vi "Triggering.vi"(11 "Test Case In":refnum<class "Test.Camera.lvclass">) -> (0 "error out":errorcluster, 3 "Test Case Out":refnum<class "Test.Camera.lvclass">)   [LabVIEW 2020, in "Test.Camera.lvclass"]
uses:
  Test.Camera.lvclass
  C:/Program Files (x86)/National Instruments/LabVIEW 2020/vi.lib/Astemes/LUnit/Test Case.lvclass
  g_industrial_cam/Camera/Camera.lvclass/Camera.ctl
  <vilib>/Astemes/LUnit/Test Case.lvclass/Test Case.ctl
  g_industrial_cam/Buffer/Buffer.lvclass/Buffer.ctl
  c3e2611f-c54f-4219-a549-b8da21c7f085.vi
  48e9c757-fedc-43ef-b150-82f816eea71f.vi
  6c7b76fd-512f-40e9-9fec-d585849d84ab.vi
  g_industrial_cam/Camera/GetSetTrigger.vi
  <vilib>/Astemes/LUnit/Append Pass Result.vi
  <vilib>/Astemes/LUnit/Append Fail Result.vi
  Get Alternative List Value.vi/1a5b698b-b1e6-4ec2-a46b-3d59f4d11909.vi
  <vilib>/Astemes/LUnit/Describe Comparison.vi
  48e9c757-fedc-43ef-b150-82f816eea71f.vi/9c5d11cd-9439-4240-a1ee-d9baace9c924.vi
  g_industrial_cam/Buffer/Access Handle.vi
  <vilib>/Astemes/LUnit/Run In UI.vi
  <vilib>/Utility/error.llb/Clear Errors.vi
  g_industrial_cam/Camera/Check Not Disconnected.vi
  <vilib>/Utility/error.llb/Error Cluster From Error Code.vi
  <vilib>/Astemes/LUnit/Describe Variant.vi
  g_industrial_cam/Camera/Destroy Stream Events.vi
  g_industrial_cam/Camera/Check Stream OK.vi
  <vilib>/Comparison/Equal/Equal Functor/Equal Functor.lvclass
  g_industrial_cam/Buffer/Buffer.lvclass
  Test.Camera.lvclass/Test.Camera.ctl
  <vilib>/Astemes/LUnit/Test Case.lvclass
  g_industrial_cam/Camera/Camera.lvclass
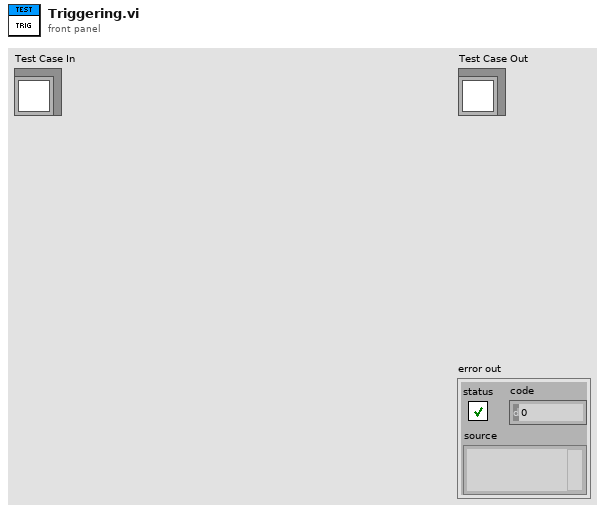
[diagram p1: front panel]
types:
  T1 = enum16{"Get Values", "Configure Trigger", "Software Trigger"}
  T2 = enum16{"Get Values", "Configure Trigger", "Software Trigger"}[]
  T3 = cluster{"Trigger Source":string, "Supported":bool, "Available Triggers":string[], "Available Trigger Sources":string[]}
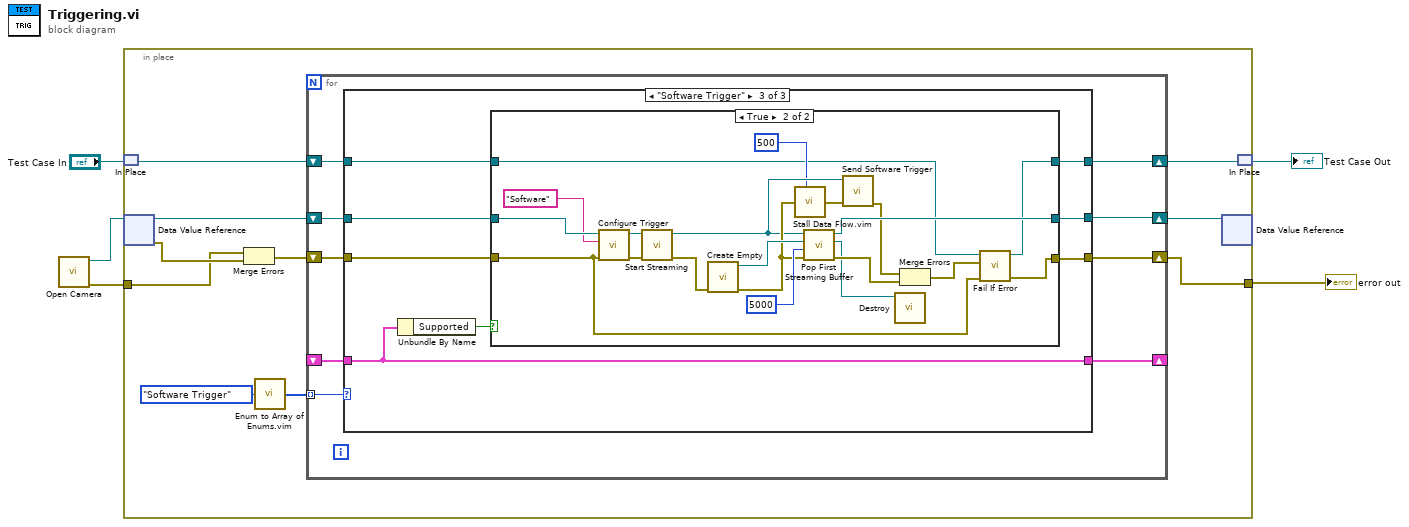
[diagram p0: block diagram]
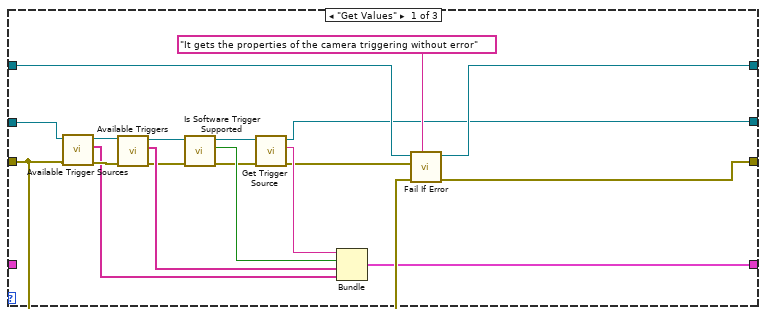
[diagram p2: hidden frame]
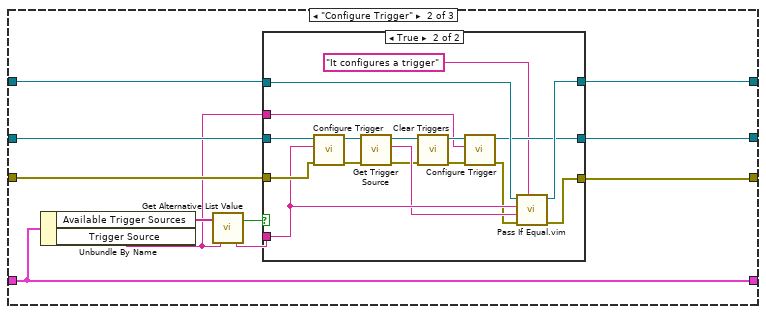
[diagram p3: hidden frame]
diagram:
  n1 = call "Open Camera.vi"() -> ("error out"=w5:errorcluster, "Camera"=w4:refnum<data-value>)  [unwired: 10 in]
  n2 = in-place {
    in-place-border: w5 -> [w8]
    in-place-border: [w7] -> w2
    n3 = in-place-match #1("Test Case In") -> (w10:refnum<class "Test.Camera.lvclass">)
    n4 = in-place-dvr #2(w4) -> (w14:refnum<class "Camera.lvclass">, w15:errorcluster)
    n5 = Merge Errors(w8, w15) -> (w13:errorcluster)
    n6 = call "Enum to Array of Enums.vim"("enum"=T1."Software Trigger") -> ("array of enums"=w11:T2)
    n7 = for {
      tunnel: w11 -> [w22] mode=indexing
      shift-right: [w21] -> w9
      shift-left: w14 -> [w24]
      shift-right: [w20] -> _
      shift-left: _ -> [w19]
      shift-right: [w17] -> w6
      shift-left: w10 -> [w18]
      shift-right: [w16] -> w7
      shift-left: w13 -> [w23]
      n8 = case shown="\"Software Trigger\"" w22 {
        tunnel: w24 -> [w38 w54 w82]
        tunnel: w23 -> [w39 w53 w81]
        tunnel: [w25 w51 w79] -> w21
        tunnel: [w28 w48 w76] -> w20
        tunnel: w19 -> [_ w48 w76]
        tunnel: w18 -> [w43 w50 w78]
        tunnel: [w42 w49 w77] -> w17
        tunnel: [w40 w52 w80] -> w16
        frame "Get Values" {
          n9 = call "Available Trigger Sources.vi"("error in (no error)"=w39, "Camera in"=w38) -> ("error out"=w37:errorcluster, "Available Trigger Sources"=w36:string[], "Camera"=w35:refnum<class "Camera.lvclass">)  [unwired: 7 in]
          n10 = call "Available Triggers.vi"("error in (no error)"=w37, "Camera in"=w35) -> ("error out"=w32:errorcluster, "Available Triggers"=w34:string[], "Camera"=w31:refnum<class "Camera.lvclass">)  [unwired: 7 in]
          n11 = call "Is Software Trigger Supported.vi"("error in (no error)"=w32, "Camera in"=w31) -> ("error out"=w30:errorcluster, "Supported"=w33:bool, "Camera"=w26:refnum<class "Camera.lvclass">)  [unwired: 7 in]
          n12 = call "Get Trigger Source.vi"("error in (no error)"=w30, "Camera in"=w26) -> ("error out"=w27:errorcluster, "Trigger Source"=w29:string, "Camera"=w25:refnum<class "Camera.lvclass">)  [unwired: 7 in]
          n13 = Bundle("Trigger Source"=w29, "Supported"=w33, "Available Triggers"=w34, "Available Trigger Sources"=w36) -> (w28:T3)  [unwired: 1 in]
          n14 = call <vilib>:"Fail If Error.vi"("Description"="It gets the properties of the camera triggering without error", "error in (no error)"=w39, "Assert error"=w27, "LUnit Test Case In"=w43) -> ("error out"=w40:errorcluster, "LUnit Test Case Out"=w42:refnum<class "Test.Camera.lvclass">)  [unwired: 6 in]
        }
        frame "Configure Trigger" {
          n15 = Unbundle By Name(w48) -> ("Available Trigger Sources"=w47:string[], "Trigger Source"=w44:string)
          n16 = call "Get Alternative List Value.vi"("Current Value"=w44, "List in"=w47) -> ("Altenative Value"=w46:string, "Alternative Available"=w45:bool)
          n17 = case shown="True" w45 {
            tunnel: w54 -> [w55 w74]
            tunnel: w53 -> [w56 w69]
            tunnel: [w56 w73] -> w52
            tunnel: [w55 w63] -> w51
            tunnel: w50 -> [w57 w71]
            tunnel: [w57 w70] -> w49
            tunnel: w46 -> [_ w66]
            tunnel: w44 -> [_ w60]
            frame False {
            }
            frame True {
              n18 = call "Configure Trigger.vi"("error in (no error)"=w69, "Source"=w66, "Camera in"=w74) -> ("error out"=w67:errorcluster, "Camera"=w72:refnum<class "Camera.lvclass">)  [unwired: 7 in]
              n19 = call "Get Trigger Source.vi"("error in (no error)"=w67, "Camera in"=w72) -> ("error out"=w62:errorcluster, "Trigger Source"=w65:string, "Camera"=w68:refnum<class "Camera.lvclass">)  [unwired: 7 in]
              n20 = call "Clear Triggers.vi"("error in (no error)"=w62, "Camera in"=w68) -> ("error out"=w61:errorcluster, "Camera"=w64:refnum<class "Camera.lvclass">)  [unwired: 8 in]
              n21 = call "Configure Trigger.vi"("error in (no error)"=w61, "Source"=w60, "Camera in"=w64) -> ("error out"=w59:errorcluster, "Camera"=w63:refnum<class "Camera.lvclass">)  [unwired: 7 in]
              n22 = call "Pass If Equal.vim"("Description"="It configures a trigger", "error in (no error)"=w59, "Actual"=w65, "Expected"=w66, "LUnit Test Case In"=w71) -> ("error out"=w73:errorcluster, "LUnit Test Case Out"=w70:refnum<class "Test.Camera.lvclass">)  [unwired: 5 in]
            }
          }
        }
        frame "Software Trigger" {
          n23 = Unbundle By Name(w76) -> ("Supported"=w75:bool)
          n24 = case shown="True" w75 {
            tunnel: w82 -> [w85 w104]
            tunnel: w81 -> [w84 w87]
            tunnel: [w84 w90] -> w80
            tunnel: [w85 w100] -> w79
            tunnel: w78 -> [w83 w89]
            tunnel: [w83 w88] -> w77
            frame False {
            }
            frame True {
              n25 = call "Configure Trigger.vi"("error in (no error)"=w87, "Source"="Software", "Camera in"=w104) -> ("error out"=w105:errorcluster, "Camera"=w102:refnum<class "Camera.lvclass">)  [unwired: 7 in]
              n26 = call "Start Streaming.vi"("error in (no error)"=w105, "Camera in"=w102) -> ("error out"=w98:errorcluster, "Camera"=w94:refnum<class "Camera.lvclass">)  [unwired: 8 in]
              n27 = call "Create Empty.vi"("error in (no error)"=w98) -> ("error out"=w96:errorcluster, "Buffer out"=w99:refnum<class "Buffer.lvclass">)  [unwired: 9 in]
              n28 = call "Stall Data Flow.vim"("value in"=w96, "milliseconds to wait"=u32 500) -> ("value out"=w95:errorcluster)  [unwired: 1 out]
              n29 = call "Pop First Streaming Buffer.vi"("error in (no error)"=w96, "Timeout (ms) Default: 10000"=5000 ("Timeout (ms) Default: -1"), "Buffer in"=w99, "Camera in"=w94) -> ("error out"=w101:errorcluster, "Buffer"=w86:refnum<class "Buffer.lvclass">, "Camera"=w100:refnum<class "Camera.lvclass">)  [unwired: 5 in]
              n30 = call "Send Software Trigger.vi"("error in (no error)"=w95, "Camera in"=w94) -> ("error out"=w91:errorcluster)  [unwired: 8 in, 1 out]
              n31 = call "Destroy.vi"("Buffer in"=w86) -> ()  [unwired: 10 in, 1 out]
              n32 = Merge Errors(w91, w101) -> (w92:errorcluster)
              n33 = call <vilib>:"Fail If Error.vi"("error in (no error)"=w87, "Assert error"=w92, "LUnit Test Case In"=w89) -> ("error out"=w90:errorcluster, "LUnit Test Case Out"=w88:refnum<class "Test.Camera.lvclass">)  [unwired: 7 in]
            }
          }
        }
      }
    }
    n34 = in-place-dvr #2(w9) -> ()  [unwired: 2 out]
    n35 = in-place-match #1(w6) -> (→"Test Case Out":refnum<class "Test.Camera.lvclass">)
  }
  "error out" <- w2
